vi "Generate Motion TA.vi"(7 "target pos mode":enum16{"backend", "frontend"}(ring), 8 "error in (no error)":errorcluster, 9 "target pos":dbl, 10 "Index":i32, 11 "Motions in":refnum<class "Motions.lvclass">) -> (0 "error out":errorcluster, 3 "Motions out":refnum<class "Motions.lvclass">)   [LabVIEW 2016, in "Hardware.lvlib" / "Motions.lvlib" / "Motions.lvclass"]
uses:
  <userlib>/Common Components/Hardware/Abstract System/Motions/Motions/Motions.lvclass
  <userlib>/Common Components/Hardware/Abstract System/Motions/Motions/Motions.lvclass/Motions.ctl
  <userlib>/Common Components/Hardware/Motor/Motor/Motor.lvclass
  <userlib>/Common Components/TriggerAction Q/TriggerAction Q/TriggerAction Q.lvclass
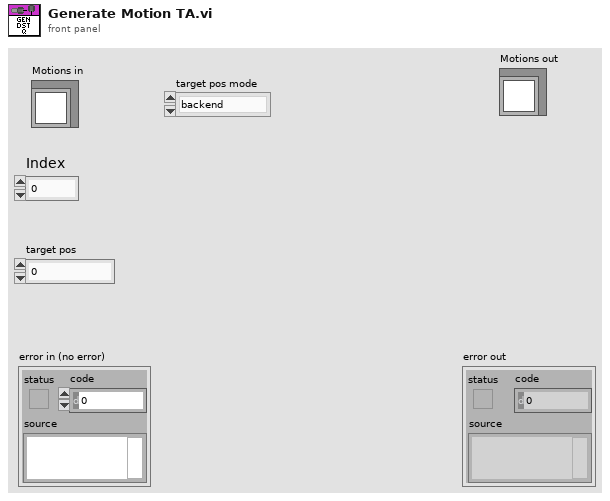
[diagram p1: front panel]
types:
  T1 = typedef "Hardware.lvlib/Motions.lvlib/Motions.lvclass/Motor States.ctl" = cluster{"Connected":bool, "Enabled":bool, "Moving Status":bool, "Soft Moving Status":bool, "Current Pos":dbl, "Target Pos":dbl, "Moving Dir (-1, 0, 1)":i32, "Error Status":bool, "Hard Limit+":bool, "Hard Limit-":bool, "Soft Limit+":bool, "Soft Limit-":bool, "History Dst Stack":refnum<queue>, "Motion Status":bool, "Motion TriggerAction Obj":refnum<class "TriggerAction Q.lvclass">}
  T2 = typedef "TriggerAction Q.lvclass/Element Data.ctl" = cluster{"Triggers":cluster{"Triggers for Array AND":string[]}[], "Actions":cluster{"Action Name":string, "Action Data":string}[]}
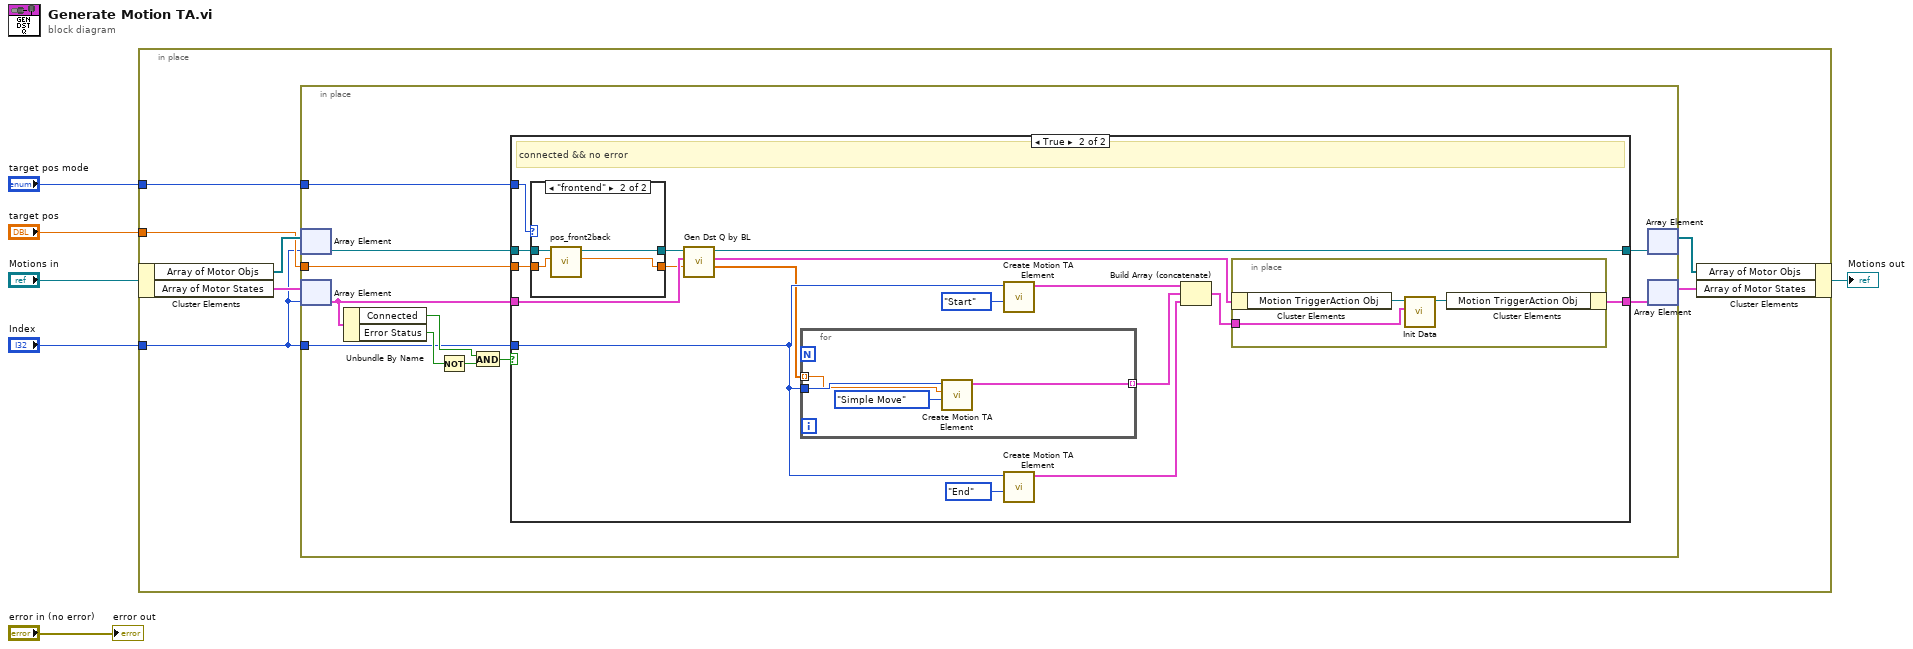
[diagram p0: block diagram]
diagram:
  n1 = in-place {
    in-place-border: "Index" -> [w7]
    in-place-border: "target pos" -> [w11]
    in-place-border: "target pos mode" -> [w8]
    n2 = in-place-cluster #1("Motions in") -> ("Array of Motor Objs"=w13:refnum<class "Motor.lvclass">[], "Array of Motor States"=w10:T1[])
    n3 = in-place {
      in-place-border: w11 -> [w23]
      in-place-border: w8 -> [w15]
      in-place-border: w7 -> [w14]
      n4 = in-place-array #2(w13, w7) -> (w24:refnum<class "Motor.lvclass">)
      n5 = in-place-array #3(w10, w7) -> (w22:T1)
      n6 = Unbundle By Name(w22) -> ("Connected"=w20:bool, "Error Status"=w19:bool)
      n7 = Not(x=w19) -> (.not. x?=w18:bool)
      n8 = And(x=w20, y=w18) -> (x .and. y?=w17:bool)
      n9 = case shown="True" w17 {
        tunnel: w24 -> [w25 w33]
        tunnel: w23 -> [_ w43]
        tunnel: w22 -> [w26 w32]
        tunnel: [w26 w41] -> w21
        tunnel: [w25 w30] -> w16
        tunnel: w15 -> [_ w42]
        tunnel: w14 -> [_ w34]
        frame False {
        }
        frame True {
          # "connected && no error"
          n10 = case shown="\"frontend\"" w42 {
            tunnel: w33 -> [w52 w56]
            tunnel: [w52 w55] -> w31
            tunnel: w43 -> [w51 w54]
            tunnel: [w51 w53] -> w28
            frame "backend", Default {
            }
            frame "frontend" {
              n11 = call <userlib>:"pos_front2back.vi"("pos frontend"=w54, "Motor in"=w56) -> ("pos backend"=w53:dbl, "Motor out"=w55:refnum<class "Motor.lvclass">)  [unwired: 7 in, 1 out]
            }
          }
          n12 = call <userlib>:"Gen Dst Q by BL.vi"("target pos (backend)"=w28, "Motor States in"=w32, "Motor Obj in"=w31) -> ("Dst Q (backend)"=w27:dbl[], "Motor States out"=w29:T1, "Motor Obj out"=w30:refnum<class "Motor.lvclass">)  [unwired: 5 in, 1 out]
          n13 = for {
            tunnel: w27 -> [w47] mode=indexing
            tunnel: [w50] -> w35 mode=indexing
            tunnel: w34 -> [w48]
            n14 = call <userlib>:"Create Motion TA Element.vi"("Option"=enum16{"Simple Move", "Start", "End"}."Simple Move", "Destination"=w47, "Index"=w48) -> ("TriggerAction element out"=w50:T2)  [unwired: 7 in, 1 out]
          }
          n15 = call <userlib>:"Create Motion TA Element.vi"("Option"=enum16{"Simple Move", "Start", "End"}."Start", "Index"=w34) -> ("TriggerAction element out"=w39:T2)  [unwired: 8 in, 1 out]
          n16 = call <userlib>:"Create Motion TA Element.vi"("Option"=enum16{"Simple Move", "Start", "End"}."End", "Index"=w34) -> ("TriggerAction element out"=w38:T2)  [unwired: 8 in, 1 out]
          n17 = Build Array (concatenate)(w39, w35, w38) -> (w40:T2[])
          n18 = in-place {
            in-place-border: w40 -> [w45]
            n19 = in-place-cluster #4(w29) -> ("Motion TriggerAction Obj"=w46:refnum<class "TriggerAction Q.lvclass">)
            n20 = call <userlib>:"Init Data.vi"("Array of TriggerAction Elements"=w45, "TriggerAction in"=w46) -> ("TriggerAction out"=w44:refnum<class "TriggerAction Q.lvclass">)  [unwired: 8 in, 1 out]
            n21 = in-place-cluster #4("Motion TriggerAction Obj"=w44) -> (w41:T1)
          }
        }
      }
      n22 = in-place-array #2(w16) -> (w12:refnum<class "Motor.lvclass">[])  [unwired: 1 out]
      n23 = in-place-array #3(w21) -> (w9:T1[])  [unwired: 1 out]
    }
    n24 = in-place-cluster #1("Array of Motor Objs"=w12, "Array of Motor States"=w9) -> (→"Motions out":refnum<class "Motions.lvclass">)
  }
  "error out" <- "error in (no error)"
